vi "OnSelect.vi"(8 "error in (no error)":errorcluster, 11 "MainMenu in":refnum<class "MainMenu.lvclass">) -> (0 "error out":errorcluster, 3 "MainMenu out":refnum<class "MainMenu.lvclass">)   [LabVIEW 2019, in "RT_Game.lvlib" / "MainMenu.lvclass"]
uses:
  MainMenu.lvclass
  Menu/Menu.lvclass
  C:/Users/FreshBob/Dropbox/VIs/myRIO_GameConsole/RT/RT_Game/Game/Game.lvclass
  Game/Game.lvclass
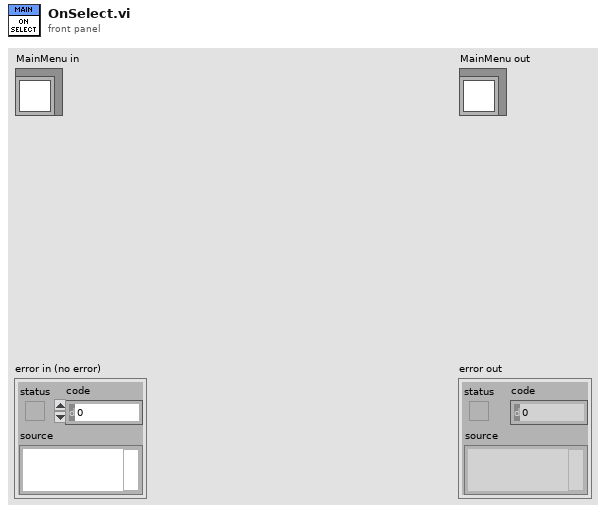
[diagram p1: front panel]
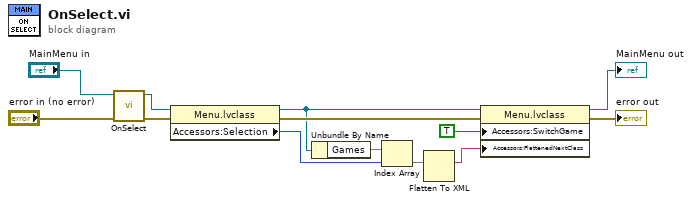
[diagram p0: block diagram]
diagram:
  n1 = call-parent "OnSelect.vi"("error in (no error)"="error in (no error)", "Menu in"="MainMenu in") -> ("error out"=w11:errorcluster, "Menu out"=w3:refnum<class "Menu.lvclass">)  [unwired: 8 in]
  n2 = property class="Menu.lvclass"(reference=w3, error in=w11) -> (reference out=w2:refnum<class "Menu.lvclass">, error out=w4:errorcluster, "Accessors:Selection"=w1:i8)
  n3 = Unbundle By Name(w2) -> ("Games"=w10)
  n4 = Index Array(array=w10, index=w1) -> (element=w6)
  n5 = Flatten To XML(anything=w6) -> (xml string=w5:string)
  n6 = property class="Menu.lvclass"(reference=w2, error in=w4, "Accessors:SwitchGame"=TRUE ("SwitchGame_"), "Accessors:FlattenedNextClass"=w5) -> (reference out=→"MainMenu out":refnum<class "Menu.lvclass">, error out=→"error out":errorcluster)
